vi "usbpt104Close.vi"(8 "error in (no error)":errorcluster, 11 "handle in":i16=16384) -> (0 "error out":errorcluster, 3 "handle out":i16)   [LabVIEW 2010]
doc: "This closes the device and should be called before exiting an application."
uses:
  UsbPT104.dll
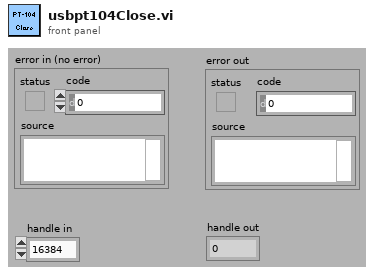
[diagram p1: front panel]
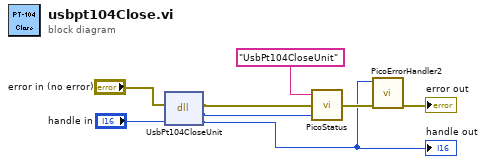
[diagram p0: block diagram]
diagram:
  n1 = dll-call lib="UsbPT104.dll" fn="UsbPt104CloseUnit"(error in="error in (no error)", "handle"="handle in") -> (error out=w3:errorcluster, "PICO_STATUS"=w1:u32, "handle"=w2:i16)  [unwired: 2 in, 1 out]
  "handle out" <- w2
  n2 = call "PicoStatus.vi"("PICO STATUS"=w1, "error in"=w3, "source"="UsbPt104CloseUnit") -> ("error out"=w8:errorcluster)
  n3 = call "PicoErrorHandler2.vi"("error in (no error)"=w8, "handle In"=w2) -> ("error out"=→"error out":errorcluster)  [unwired: 9 in]
